vi "FPGA-TrapTest-05-2017.vi"() -> ()   [LabVIEW 2010]
uses:
  <vilib>/eio/EIONode/EIONode.xnode
  <vilib>/rvi/eio/nirviEIOImplementation/nirviEIOImplementation.xnode
  <vilib>/rvi/eio/common/nirviEmuClasses.ctl
  <vilib>/rvi/eio/common/nirviEmuTemplateMethod_noerrors.vi
panel:
  out "MainCol2b":fxp<+/-,26,5> format="%.23g"
  out "MainCol2a":fxp<+/-,26,5> format="%.23g"
  out "MainCol1b":fxp<+/-,26,5> format="%.23g"
  out "MainCol1a":fxp<+/-,26,5> format="%.23g"
  out "PreCol2":fxp<+/-,26,5> format="%.23g"
  out "PreCol1":fxp<+/-,26,5> format="%.23g"
  out "MesswertTrap2":fxp<+/-,27,6> format="%.23g"
  in  "PIDTrap2":T1={"proportional gain (Kc)"=1.0, "integral gain (Kc*Ts/Ti)"=1.66796875, "derivative gain (Kc*Td/Ts)"=0.0} {"proportional gain (Kc)" format="%.11g"; "integral gain (Kc*Ts/Ti)" format="%.11g"; "derivative gain (Kc*Td/Ts)" format="%.11g"}
  in  "setpointTrap2":fxp<+/-,16,6> format="%.12g"
  in  "HeizenTrap2":bool
  out "Thermoelement":fxp<+/-,26,5> format="%.23g"
  out "PTStirling":fxp<+/-,26,5> format="%.23g"
  in  "Stirling":bool
  in  "stop":bool
  in  "setpointTrap1":fxp<+/-,16,6> format="%.12g"
  in  "Messwerte":i32
  in  "HeizenTrap1":bool
  in  "5Van(us)":u16
  in  "Periode(us)":u32
  out "MesswertTrap1":fxp<+/-,27,6> format="%.23g"
  in  "Warten(us)":u16
  in  "zwischenMesswerten(us)":u16
  in  "PIDTrap1":T1={"proportional gain (Kc)"=1.0, "integral gain (Kc*Ts/Ti)"=1.66796875, "derivative gain (Kc*Td/Ts)"=0.0} {"proportional gain (Kc)" format="%.11g"; "integral gain (Kc*Ts/Ti)" format="%.11g"; "derivative gain (Kc*Td/Ts)" format="%.11g"}
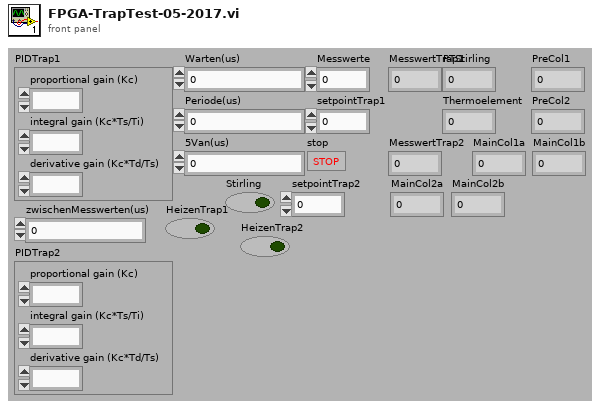
[diagram p1: front panel]
types:
  T1 = cluster{"proportional gain (Kc)":fxp<+/-,16,8>, "integral gain (Kc*Ts/Ti)":fxp<+/-,16,8>, "derivative gain (Kc*Td/Ts)":fxp<+/-,16,8>}
  T2 = typedef "nirviEmuClasses.ctl" = enum16{"IO Read", "IO Write", "Method", "Property Read", "Property Write"}
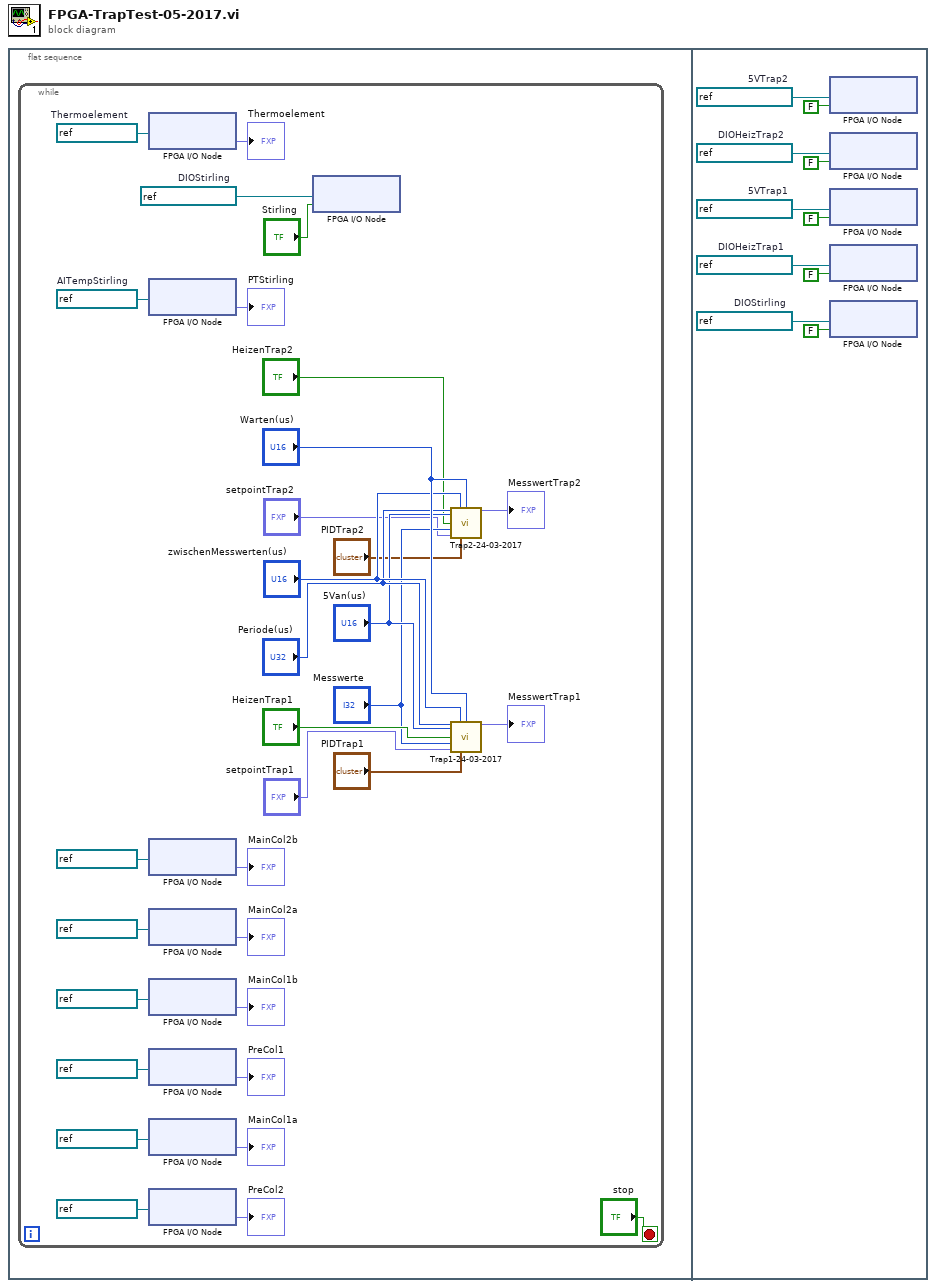
[diagram p0: block diagram]
diagram:
  n1 = flat-sequence {
    frame #0 {
      n2 = while {
        stop <- "stop" stop-if-true
        w27 = refnum<k21> "Mod1/AI3"  # Thermoelement
        w29 = refnum<k21> "Mod1/AI2"  # AITempStirling
        w31 = refnum<k21> "Mod6/DIO12"  # DIOStirling
        n3 = xnode "FPGA I/O Node"("FPGA I/O In"=w27) -> ("I/O Item"=→"Thermoelement":fxp<+/-,26,5>)  [unwired: 1 out]
        n4 = xnode "FPGA I/O Node"("FPGA I/O In"=w29) -> ("I/O Item"=→"PTStirling":fxp<+/-,26,5>)  [unwired: 1 out]
        n5 = xnode "FPGA I/O Node"("FPGA I/O In"=refnum<k21> "Mod1/AI8") -> ("I/O Item"=→"MainCol2b":fxp<+/-,26,5>)  [unwired: 1 out]
        n6 = xnode "FPGA I/O Node"("FPGA I/O In"=refnum<k21> "Mod1/AI7") -> ("I/O Item"=→"MainCol2a":fxp<+/-,26,5>)  [unwired: 1 out]
        n7 = xnode "FPGA I/O Node"("FPGA I/O In"=refnum<k21> "Mod1/AI6") -> ("I/O Item"=→"MainCol1b":fxp<+/-,26,5>)  [unwired: 1 out]
        n8 = xnode "FPGA I/O Node"("FPGA I/O In"=refnum<k21> "Mod1/AI3") -> ("I/O Item"=→"PreCol1":fxp<+/-,26,5>)  [unwired: 1 out]
        n9 = xnode "FPGA I/O Node"("FPGA I/O In"=refnum<k21> "Mod1/AI5") -> ("I/O Item"=→"MainCol1a":fxp<+/-,26,5>)  [unwired: 1 out]
        n10 = xnode "FPGA I/O Node"("FPGA I/O In"=refnum<k21> "Mod1/AI4") -> ("I/O Item"=→"PreCol2":fxp<+/-,26,5>)  [unwired: 1 out]
        n11 = xnode "FPGA I/O Node"("I/O Item"="Stirling", "FPGA I/O In"=w31) -> ()  [unwired: 1 out]
        n12 = call "Trap2-24-03-2017.vi"("Periode(us)"="Periode(us)", "zwischenMesswerten(us)"="zwischenMesswerten(us)", "Warten(us)"="Warten(us)", "5Van(us)"="5Van(us)", "Heizen"="HeizenTrap2", "Messwerte"="Messwerte", "setpoint"="setpointTrap2", "PID gains"="PIDTrap2") -> ("Messwert"=→"MesswertTrap2":fxp<+/-,27,6>)  [unwired: 7 in]
        n13 = call "Trap1-24-03-2017.vi"("Periode(us)"="Periode(us)", "zwischenMesswerten(us)"="zwischenMesswerten(us)", "Warten(us)"="Warten(us)", "5Van(us)"="5Van(us)", "Heizen"="HeizenTrap1", "Messwerte"="Messwerte", "setpoint"="setpointTrap1", "PID gains"="PIDTrap1") -> ("Messwert"=→"MesswertTrap1":fxp<+/-,27,6>)  [unwired: 7 in]
      }
    }
    frame #1 {
      w197 = refnum<k21> "Mod6/DIO18"  # DIOHeizTrap2
      w199 = refnum<k21> "Mod6/DIO20"  # 5VTrap2
      w201 = refnum<k21> "Mod6/DIO12"  # DIOStirling
      w203 = refnum<k21> "Mod6/DIO19"  # DIOHeizTrap1
      w205 = refnum<k21> "Mod6/DIO21"  # 5VTrap1
      n14 = xnode "FPGA I/O Node"("I/O Item"=FALSE, "FPGA I/O In"=w199) -> ()  [unwired: 1 out]
      n15 = xnode "FPGA I/O Node"("I/O Item"=FALSE, "FPGA I/O In"=w197) -> ()  [unwired: 1 out]
      n16 = xnode "FPGA I/O Node"("I/O Item"=FALSE, "FPGA I/O In"=w205) -> ()  [unwired: 1 out]
      n17 = xnode "FPGA I/O Node"("I/O Item"=FALSE, "FPGA I/O In"=w203) -> ()  [unwired: 1 out]
      n18 = xnode "FPGA I/O Node"("I/O Item"=FALSE, "FPGA I/O In"=w201) -> ()  [unwired: 1 out]
    }
  }
